vi "midiOutPlayer.Launch.vi"(8 "error in":errorcluster, 10 "MIDI Events":T1(array[cluster]), 11 "midi in":refnum<class "midi.lvclass">) -> (0 "error out":errorcluster, 3 "midi out":refnum<class "midi.lvclass">)   [LabVIEW 2020, in "midi.lvclass"]
uses:
  midi.lvclass
  midi.lvclass/midi.ctl
  midiOutPlayer.Core.vi
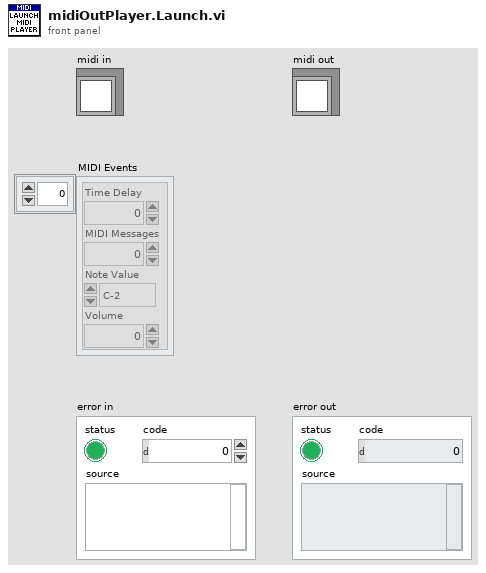
[diagram p1: front panel]
types:
  T1 = cluster{"Time Delay":u32, "MIDI Messages":u16, "Note Value":enum8{"C-2", "C#-2", "D-2", "D#-2", "E-2", "F-2", "F#-2", "G-2", "G#-2", "A-2", "A#-2", "B-2", "C-1", "C#-1", "D-1", "D#-1", "E-1", "F-1", "F#-1", "G-1", "G#-1", "A-1", "A#-1", "B-1", "C0", "C#0", "D0", "D#0", "E0", "F0", "F#0", "G0", "G#0", "A0", "A#0", "B0", "C1", "C#1", "D1", "D#1", "E1", "F1", "F#1", "G1", "G#1", "A1", "A#1", "B1", "C2", "C#2", "D2", "D#2", "E2", "F2", "F#2", "G2", "G#2", "A2", "A#2", "B2", "C3", "C#3", "D3", "D#3", "E3", "F3", "F#3", "G3", "G#3", "A3", "A#3", "B3", "C4", "C#4", "D4", "D#4", "E4", "F4", "F#4", "G4", "G#4", "A4", "A#4", "B4", "C5", "C#5", "D5", "D#5", "E5", "F5", "F#5", "G5", "G#5", "A5", "A#5", "B5", "C6", "C#6", "D6", "D#6", "E6", "F6", "F#6", "G6", "G#6", "A6", "A#6", "B6", "C7", "C#7", "D7", "D#7", "E7", "F7", "F#7", "G7", "G#7", "A7", "A#7", "B7", "C8", "C#8", "D8", "D#8", "E8", "F8", "F#8", "G"}, "Volume":u8}[]
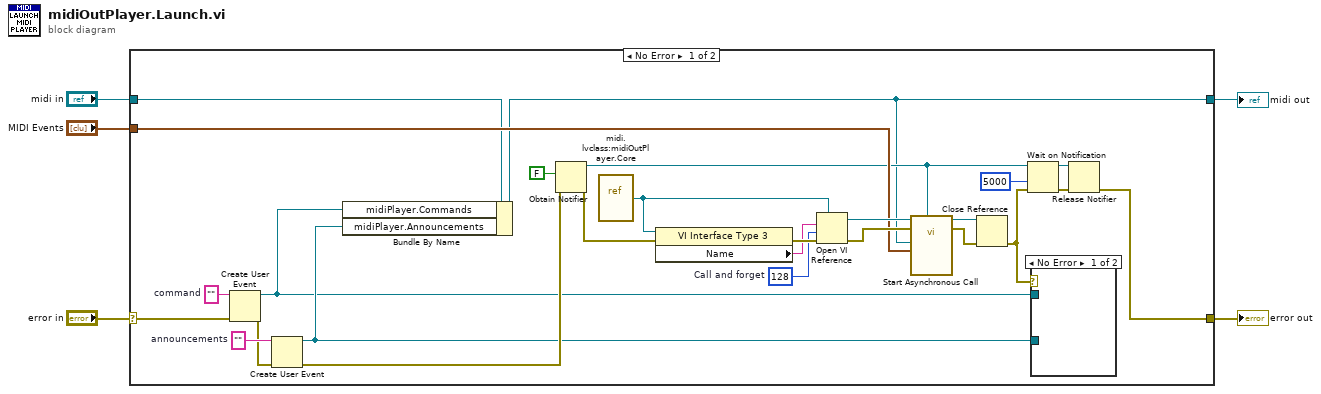
[diagram p0: block diagram]
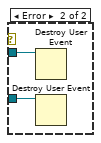
[diagram p2: hidden frame]
diagram:
  n1 = case shown="No Error" "error in" {
    selector: "error in" -> [w23 w35]
    tunnel: [w6 w35] -> w4
    tunnel: "midi in" -> [w10 w34]
    tunnel: "MIDI Events" -> [w21 _]
    tunnel: [w9 w34] -> w1
    frame No Error {
      w18 = ""  # announcements
      w22 = 128  # Call and forget
      w31 = ""  # command
      n2 = Create User Event(user event datatype=w31, error in=w23) -> (user event=w7:refnum<user-event>, error out=w17:errorcluster)
      n3 = Create User Event(user event datatype=w18, error in=w17) -> (user event=w8:refnum<user-event>, error out=w16:errorcluster)
      n4 = Bundle By Name(cluster=w10, "midiPlayer.Commands"=w7, "midiPlayer.Announcements"=w8) -> (w9:refnum<class "midi.lvclass">)
      n5 = Obtain Notifier(notification data type=FALSE, error in (no error)=w16) -> (notifier out=w15:refnum<notifier>, error out=w24:errorcluster)  [unwired: 2 in, 1 out]
      n6 = vi-ref "midi.lvclass:midiOutPlayer.Core.vi"() -> (w27:refnum<vi>)
      n7 = property class="VI Interface Type 3"(reference=w27, error in=w24) -> (error out=w26:errorcluster, "Name"=w25:string)  [unwired: 1 out]
      n8 = Open VI Reference(type specifier VI Refnum (for type only)=w27, vi path=w25, options=w22, error in (no error)=w26) -> (vi reference=w28:refnum<vi>, error out=w29:errorcluster)  [unwired: 2 in]
      n9 = call-by-ref "Start Asynchronous Call"(reference=w28, error in=w29, "notifier out"=w15, "MIDI Events"=w21, "midi out"=w9) -> (reference out=w20:refnum<vi>, error out=w19:errorcluster)  [unwired: 9 in]
      n10 = Close Reference(reference=w20, error in (no error)=w19) -> (error out=w14:errorcluster)
      n11 = Wait on Notification(notifier=w15, timeout in ms (-1)=5000, error in (no error)=w14) -> (notifier out=w13:refnum<notifier>, error out=w12:errorcluster)  [unwired: 1 in, 2 out]
      n12 = case shown="No Error" w14 {
        tunnel: w7 -> [_ w33]
        tunnel: w8 -> [_ w32]
        frame No Error {
        }
        frame Error {
          n13 = Destroy User Event(user event=w33) -> ()  [unwired: 1 in, 1 out]
          n14 = Destroy User Event(user event=w32) -> ()  [unwired: 1 in, 1 out]
        }
      }
      n15 = Release Notifier(notifier=w13, error in (no error)=w12) -> (error out=w6:errorcluster)  [unwired: 1 in, 2 out]
    }
    frame Error {
    }
  }
  "error out" <- w4
  "midi out" <- w1
